vi "View Holder.vi"(8 "error in (no error)":errorcluster, 11 "View In":refnum<class "View.lvclass">) -> (0 "error out":errorcluster)   [LabVIEW 2020, in "View.lvclass"]
uses:
  View.lvclass
  View.lvclass/View.ctl
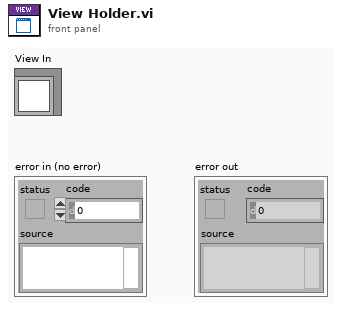
[diagram p1: front panel]
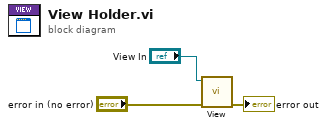
[diagram p0: block diagram]
diagram:
  n1 = call-dynamic "View.vi"("error in (no error)"="error in (no error)", "View In"="View In") -> ("error out"=→"error out":errorcluster)  [unwired: 9 in]
